vi "How a Case works.vi"() -> ()   [LabVIEW 2012]
uses:
  <vilib>/rvi/FXPMathLib/basic elements/FxpIntAccumulator/subVIs/nifxpmath_IntAccumulator_SimConfig.ctl
  <vilib>/rvi/FXPMathLib/basic elements/FxpIntAccumulator/simVIs/DllFxpIntAccumulator_sub.vi
  <vilib>/rvi/FXPMathLib/basic elements/FxpIntAccumulator/XNode/nifxpmath_IntAccumulator.xnode
panel:
  out "Accumulator Output":dbl
  in  "Accumulator Input":dbl
  out "Slide":dbl(slide) scale=0.0..10.0
  out "Boolean 6":bool
  out "Boolean 5":bool
  in  "Numeric 5":i32
  in  "Numeric 4":i32
  out "Boolean 4":bool
  in  "Boolean 3":bool
  in  "Boolean 2":bool
  in  "Boolean":bool
  out "Numeric 3":dbl
  out "Numeric 2":dbl
  out "3":bool
  out "2":bool
  out "1":bool
  in  "Numeric":i32
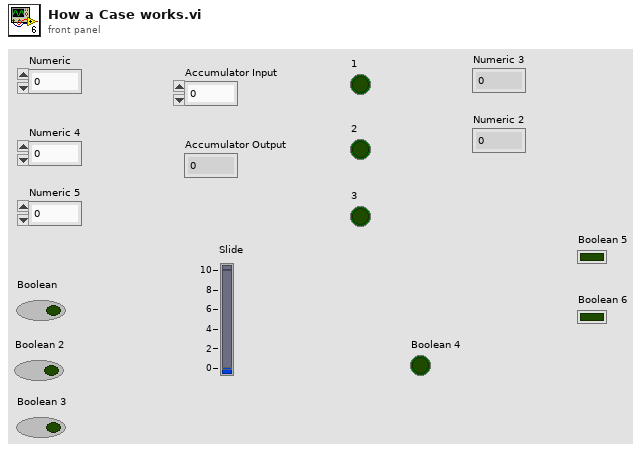
[diagram p1: front panel]
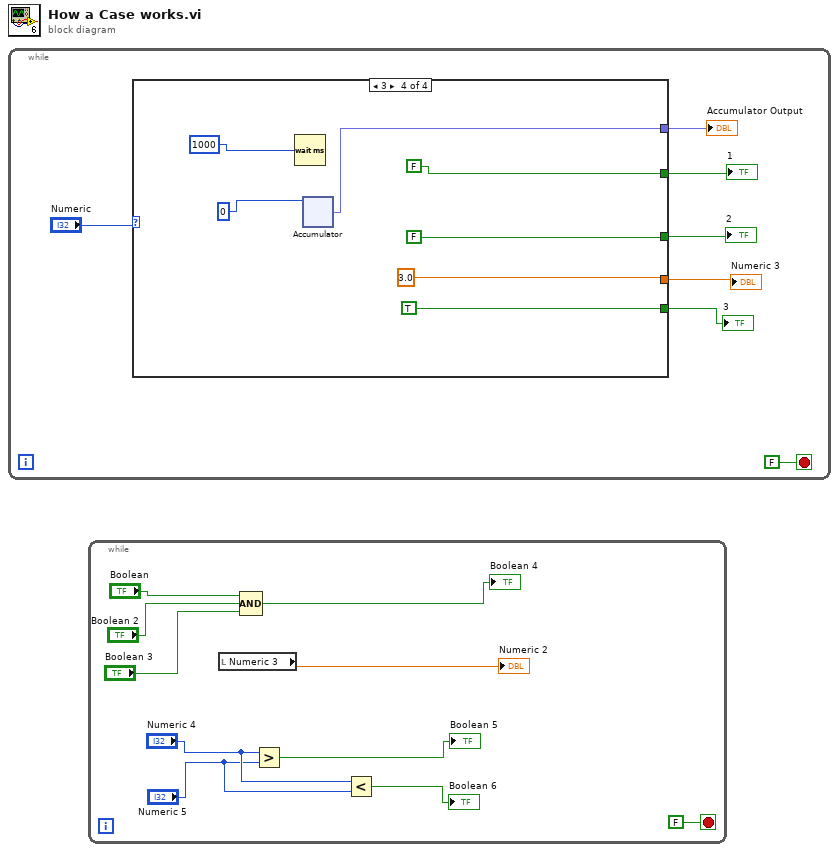
[diagram p0: block diagram]
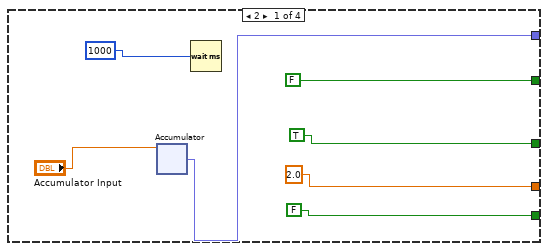
[diagram p2: hidden frame]
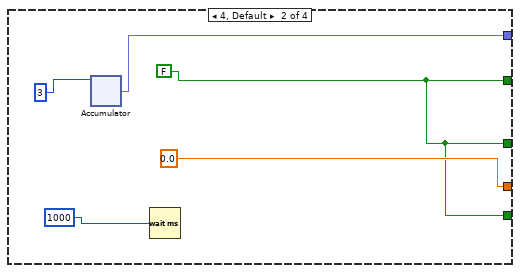
[diagram p3: hidden frame]
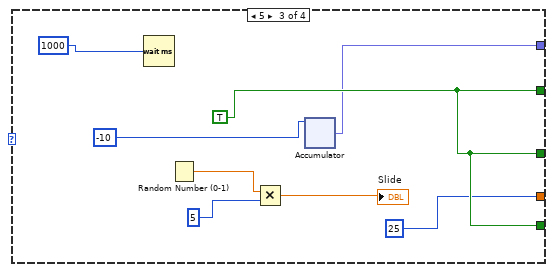
[diagram p4: hidden frame]
diagram:
  n1 = while {
    stop <- FALSE stop-if-true
    n2 = case shown="3" "Numeric" {
      tunnel: [FALSE w45 w78 TRUE] -> w6
      tunnel: [TRUE w45 w78 FALSE] -> w5
      tunnel: [FALSE w45 w78 FALSE] -> w4
      tunnel: [2.0 0.0 25 3.0] -> w2
      tunnel: [w8 w43 w71 w104] -> w1
      frame 2 {
        n3 = xnode "Accumulator"("x"="Accumulator Input") -> ("s"=w8:fxp<+,64,38>)  [unwired: 4 in, 1 out]
        n4 = Wait (ms)(milliseconds to wait=1000) -> ()  [unwired: 1 out]
      }
      frame 4, Default {
        w45 = FALSE
        n5 = xnode "Accumulator"("x"=3) -> ("s"=w43:fxp<+/-,64,64>)  [unwired: 4 in, 1 out]
        n6 = Wait (ms)(milliseconds to wait=1000) -> ()  [unwired: 1 out]
      }
      frame 5 {
        w78 = TRUE
        n7 = Wait (ms)(milliseconds to wait=1000) -> ()  [unwired: 1 out]
        n8 = Random Number (0-1)() -> (number: 0 to 1=w76:dbl)
        n9 = Multiply(x=w76, y=5) -> (x*y=→"Slide":dbl)
        n10 = xnode "Accumulator"("x"=-10) -> ("s"=w71:fxp<+/-,64,64>)  [unwired: 4 in, 1 out]
      }
      frame 3 {
        n11 = Wait (ms)(milliseconds to wait=1000) -> ()  [unwired: 1 out]
        n12 = xnode "Accumulator"("x"=0) -> ("s"=w104:fxp<+/-,64,64>)  [unwired: 4 in, 1 out]
      }
    }
    "1" <- w4
    "2" <- w5
    "3" <- w6
    "Numeric 3" <- w2
    "Accumulator Output" <- w1
  }
  n13 = while {
    stop <- FALSE stop-if-true
    n14 = local read "Numeric 3"() -> (→"Numeric 2":dbl)
    n15 = Compound Arithmetic op=AND("Boolean", "Boolean 2", "Boolean 3") -> (→"Boolean 4":bool)
    n16 = Greater?(x="Numeric 4", y="Numeric 5") -> (0:→"Boolean 5":bool)
    n17 = Less?(x="Numeric 4", y="Numeric 5") -> (x < y?=→"Boolean 6":bool)
  }
